vi "数据查询_数据查询_古田污水厂.vi"() -> ()   [LabVIEW 2016]
uses:
  <vilib>/Utility/miscctls.llb/LVPointTypeDef.ctl
  <vilib>/Utility/miscctls.llb/LVRowAndColumnUnsignedTypeDef.ctl
  <vilib>/addons/database/_DB Variant To Data/Database Variant To Data.xnode
panel:
  in  "工作模式":string(combo)="全部数据"
  out "连接的字符串":string
  out "选中数据表":string
  in  "查询":bool
  in  "结束日期":string="2020/01/01"
  in  "起始日期":string="2010/01/01"
  out "XY图":cluster{"data":timestamp[], "data":dbl[]}[](graph)
  in  "组合框":string(combo)
  out "数据表":string[][](table)
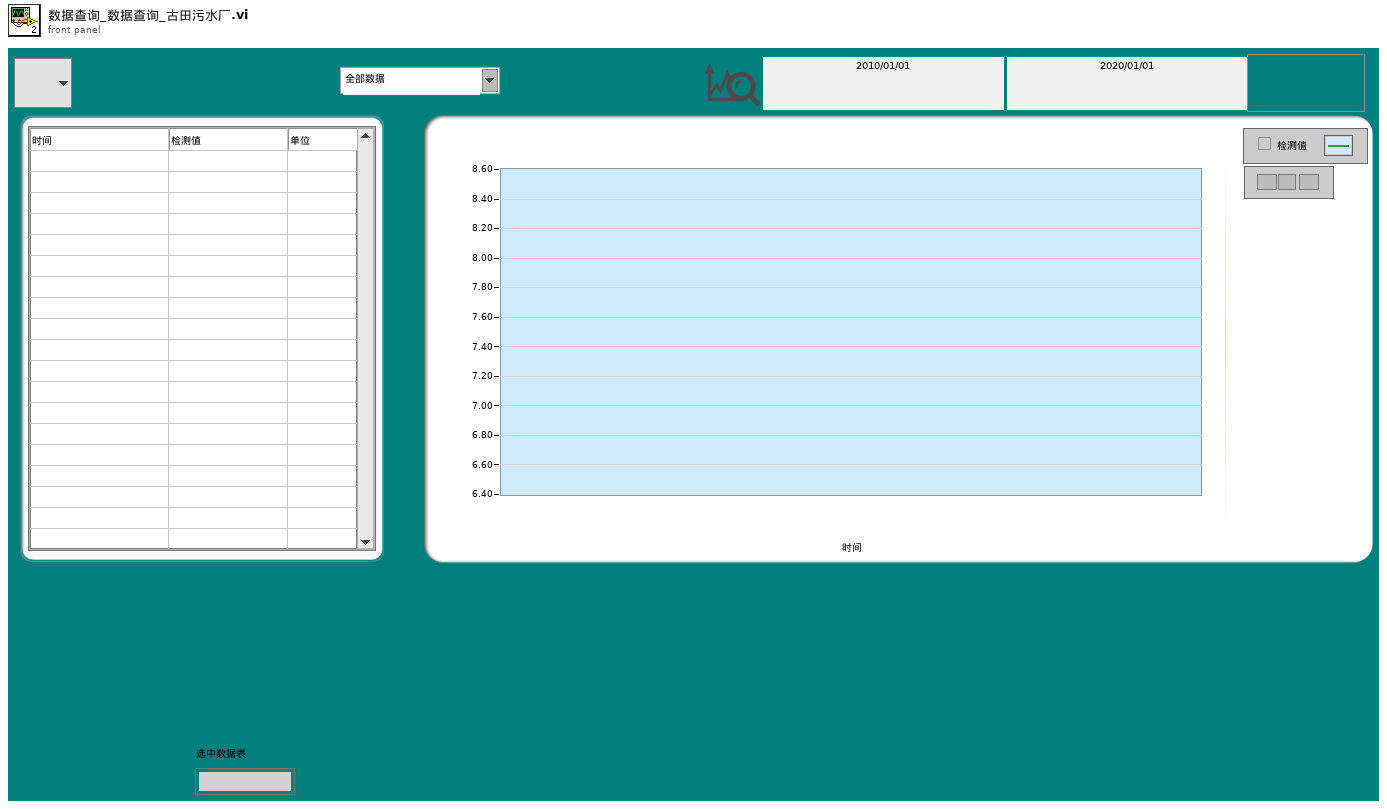
[diagram p1: front panel]
types:
  T1 = typedef "LVPointTypeDef.ctl" = cluster{"Horizontal":i16, "Vertical":i16}
  T2 = typedef "LVRowAndColumnUnsignedTypeDef.ctl" = cluster{"Row":u32, "Column":u32}
  T3 = typedef "LVPoint32TypeDef.ctl" = cluster{"Horizontal":i32, "Vertical":i32}
  T4 = typedef "LVPointDoubleTypeDef.ctl" = cluster{"Cursor X":dbl, "Cursor Y":dbl}
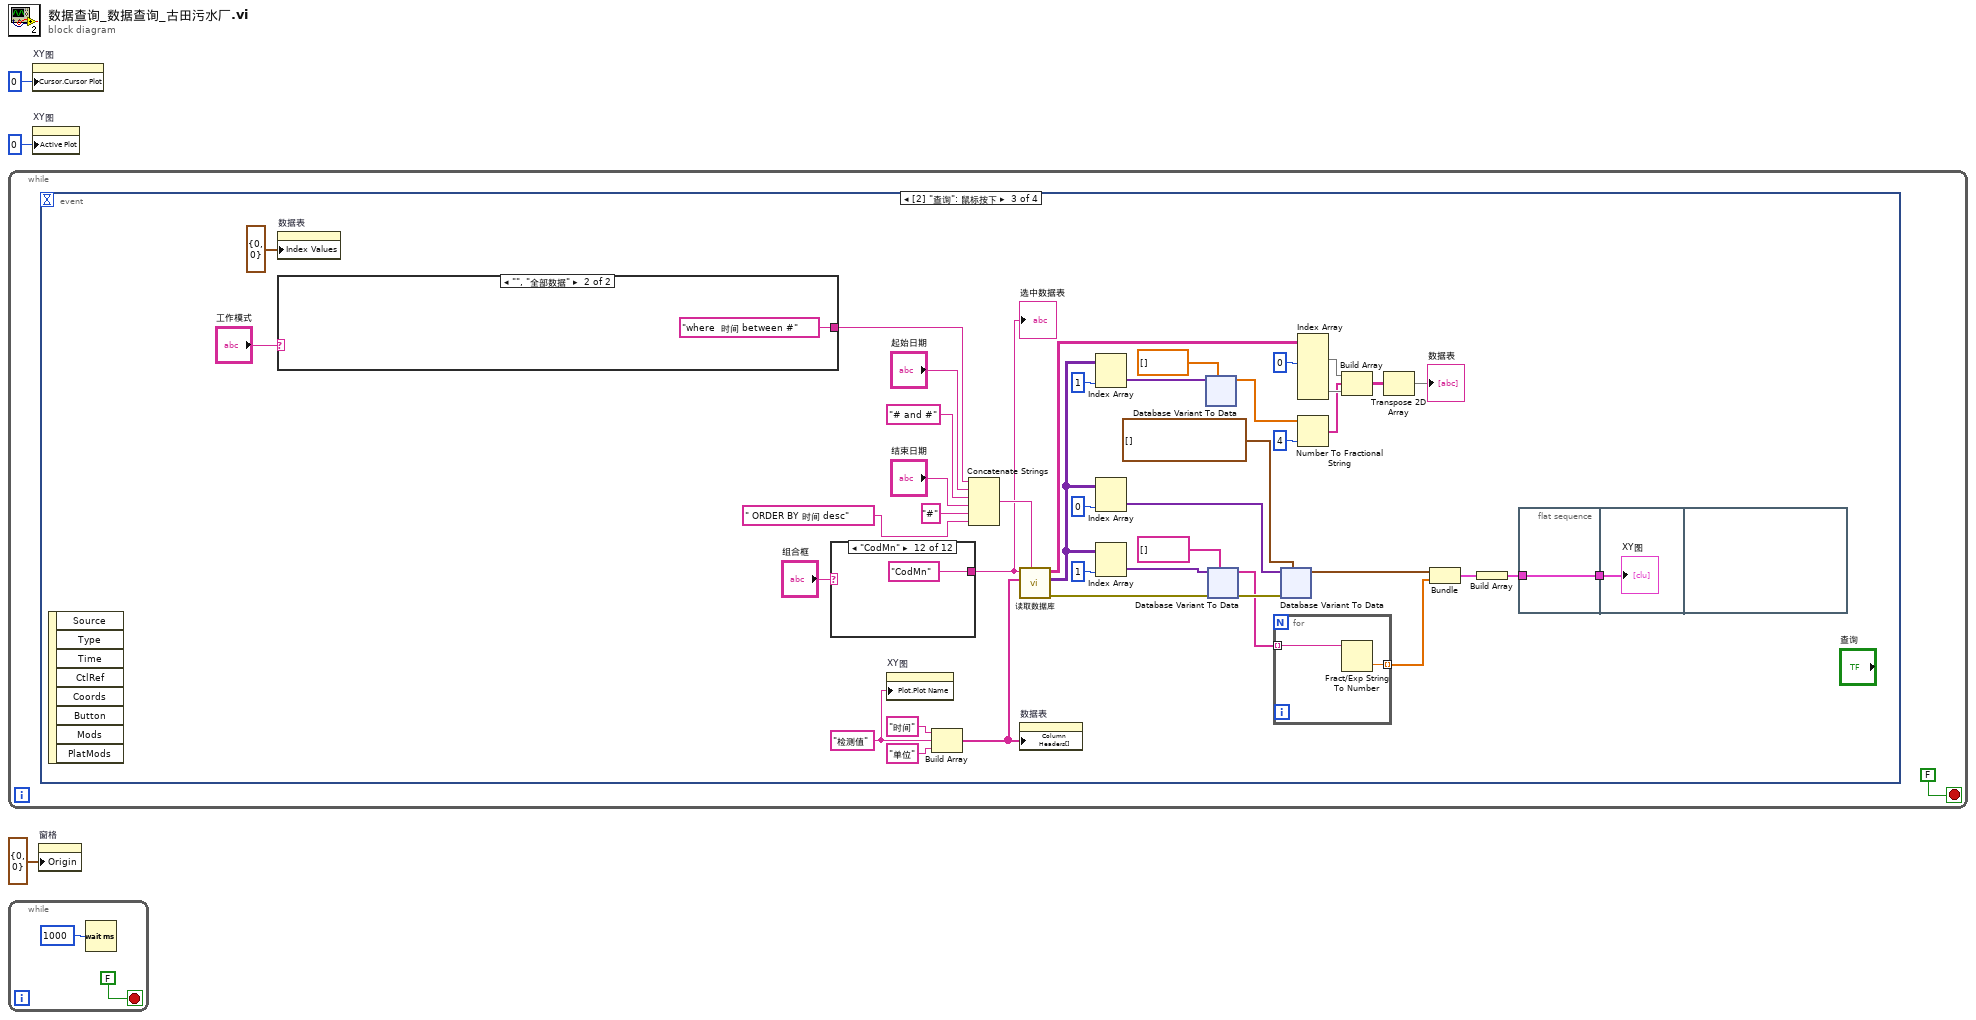
[diagram p0: block diagram]
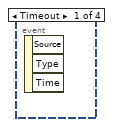
[diagram p2: hidden frame]
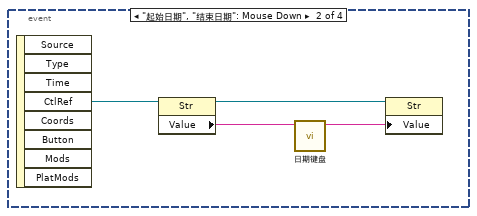
[diagram p3: hidden frame]
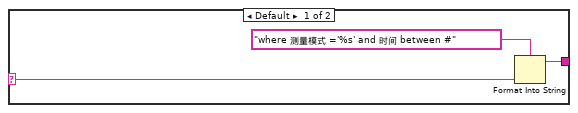
[diagram p4: hidden frame]
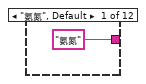
[diagram p5: hidden frame]
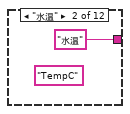
[diagram p6: hidden frame]
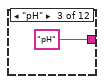
[diagram p7: hidden frame]
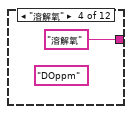
[diagram p8: hidden frame]
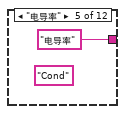
[diagram p9: hidden frame]
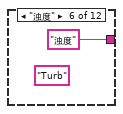
[diagram p10: hidden frame]
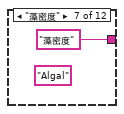
[diagram p11: hidden frame]
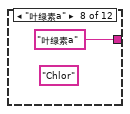
[diagram p12: hidden frame]
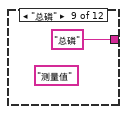
[diagram p13: hidden frame]
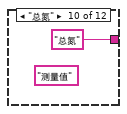
[diagram p14: hidden frame]
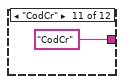
[diagram p15: hidden frame]
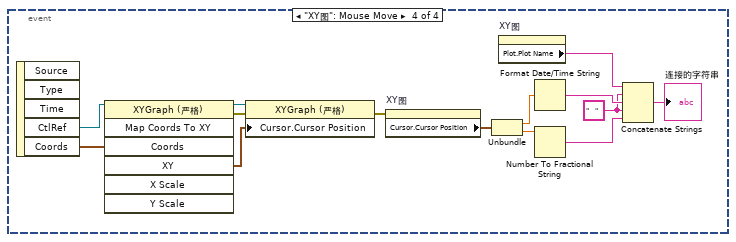
[diagram p16: hidden frame]
diagram:
  n1 = while {
    stop <- FALSE stop-if-true
    n2 = event shown="[2] \"查询\": 鼠标按下" {
      selector: _ -> [_ _ _ _]
      dyn-events: _ -> [_ _ _ _]
      timeout: _ -> [_ _ _ _]
      event Timeout {
        n3 = event-data() -> ()  [unwired: 1 in, 3 out]
      }
      event "起始日期", "结束日期": Mouse Down {
        n4 = event-data() -> ("CtlRef"=w8:refnum<vi>)  [unwired: 1 in, 7 out]
        n5 = property class="Str"(reference=w8) -> (reference out=w6:refnum<vi>, "Value"=w7:string)  [unwired: 1 in, 1 out]
        n6 = call "日期键盘.vi"("原值"=w7) -> ("x+y"=w5:string)  [unwired: 10 in]
        n7 = property class="Str"(reference=w6, "Value"=w5) -> ()  [unwired: 1 in, 2 out]
      }
      event "查询": Mouse Down {
        w22 = "检测值"
        n8 = event-data() -> ()  [unwired: 1 in, 8 out]
        n9 = property on="数据表" class="Tbl (严格)"("Index Values"=T2 {"Row"=0, "Column"=0} ("索引值")) -> ()  [unwired: 2 in, 2 out]
        n10 = case shown="\"\", \"全部数据\"" "工作模式" {
          selector: "工作模式" -> [w53 _]
          tunnel: [w51 "where  时间 between #" ("condition")] -> w10
          frame Default {
            n11 = Format Into String(format string="where 测量模式 ='%s' and 时间 between #" ("condition"), w53) -> (resulting string=w51:string)  [unwired: 2 in, 1 out]
          }
          frame "", "全部数据" {
          }
        }
        n12 = case shown="\"CodMn\"" "组合框" {
          tunnel: ["氨氮" "水温" "pH" "溶解氧" "电导率" "浊度" "藻密度" "叶绿素a" "总磷" "总氮" "CodCr" "CodMn"] -> w24
          frame "氨氮", Default {
          }
          frame "水温" {
            (unwired) "TempC"
          }
          frame "pH" {
          }
          frame "溶解氧" {
            (unwired) "DOppm"
          }
          frame "电导率" {
            (unwired) "Cond"
          }
          frame "浊度" {
            (unwired) "Turb"
          }
          frame "藻密度" {
            (unwired) "Algal"
          }
          frame "叶绿素a" {
            (unwired) "Chlor"
          }
          frame "总磷" {
            (unwired) "测量值"
          }
          frame "总氮" {
            (unwired) "测量值"
          }
          frame "CodCr" {
          }
          frame "CodMn" {
          }
        }
        "选中数据表" <- w24
        n13 = property on="XY图" class="XYGraph (严格)"("Plot.Plot Name"=w22) -> ()  [unwired: 2 in, 2 out]
        n14 = Build Array("时间", w22, "单位" ("元素")) -> (w25:string[])
        n15 = Concatenate Strings(w10, "起始日期", "# and #" ("condition"), "结束日期", "#" ("condition"), " ORDER BY 时间 desc" ("字符串")) -> (w49:string)
        n16 = call "读取数据库.vi"("condition"=w49, "显示项"=w25, "组合框"=w24) -> ("error out"=w40:errorcluster, "data"=w19:variant[][], "表格"=w32:string[][])  [unwired: 5 in, 1 out]
        n17 = property on="数据表" class="Tbl (严格)"("Column Headers[]"=w25) -> ()  [unwired: 2 in, 2 out]
        n18 = Index Array(array=w19, index (col)=1 ("禁用的索引 (列)")) -> (element=w17:variant[])  [unwired: 1 in]
        n19 = Index Array(array=w19, index (col)=0 ("禁用的索引 (列)")) -> (element=w43:variant[])  [unwired: 1 in]
        n20 = Index Array(array=w19, index (col)=1 ("禁用的索引 (列)")) -> (element=w41:variant[])  [unwired: 1 in]
        n21 = xnode "Database Variant To Data"("database variant"=w17, "type"=sgl[] []) -> ("data"=w15:sgl[])  [unwired: 1 in, 1 out]
        n22 = xnode "Database Variant To Data"("database variant"=w41, "error in (no error)"=w40, "type"=string[] []) -> ("data"=w23:string[], "error out"=w39:errorcluster)
        n23 = for {
          tunnel: w23 -> [w94] mode=indexing
          tunnel: [w93] -> w9 mode=indexing
          n24 = Fract/Exp String To Number(string=w94) -> (number=w93:dbl)  [unwired: 3 in, 1 out]
        }
        n25 = xnode "Database Variant To Data"("database variant"=w43, "error in (no error)"=w39, "type"=timestamp[] []) -> ("data"=w34:timestamp[])  [unwired: 1 out]
        n26 = Index Array(array=w32, index (col) #1=0 ("禁用的索引 (列)")) -> (element #1=w30:string[], element #3=w20:string[])  [unwired: 5 in, 1 out]
        n27 = Number To Fractional String(number=w15, precision (6)=i16 4 ("精度(6)")) -> (F-format string=w13:string[])  [unwired: 2 in]
        n28 = Build Array(w30, w13, w20) -> (w29:string[][])
        n29 = Transpose 2D Array(2D array=w29) -> (transposed array=→"数据表":string[][])
        n30 = Bundle("data"=w34, w9) -> (w35:cluster{"data":timestamp[], dbl[]})  [unwired: 1 in]
        n31 = Build Array(w35) -> (w36:cluster{"data":timestamp[], dbl[]}[])
        n32 = flat-sequence {
          tunnel: [w107] -> w37
          tunnel: w36 -> [w107]
          tunnel: w37 -> [w108]
          frame #0 {
          }
          frame #1 {
            "XY图" <- w108
          }
          frame #2 {
          }
        }
      }
      event "XY图": Mouse Move {
        w202 = "   " ("字符串")
        n33 = event-data() -> ("CtlRef"=w212:refnum<vi>, "Coords"=w211:T3)  [unwired: 1 in, 3 out]
        n34 = invoke class="XYGraph (严格)" method="Map Coords To XY"(reference=w212, "Coords"=w211) -> (reference out=w210:refnum<vi>, error out=w207:errorcluster, "XY"=w209:cluster{"X":dbl, "Y":dbl})  [unwired: 5 in, 4 out]
        n35 = property class="XYGraph (严格)"(reference=w210, error in=w207, "Cursor.Cursor Position"=w209) -> (error out=w208:errorcluster)  [unwired: 1 out]
        n36 = property on="XY图" class="XYGraph (严格)"(error in=w208) -> ("Cursor.Cursor Position"=w205:T4)  [unwired: 1 in, 2 out]
        n37 = Unbundle(w205) -> ("Cursor X"=w204:dbl, "Cursor Y"=w201:dbl)
        n38 = property on="XY图" class="XYGraph (严格)"() -> ("Plot.Plot Name"=w199:string)  [unwired: 2 in, 2 out]
        n39 = Format Date/Time String(seconds (now)=w204) -> (date/time string=w203:string)  [unwired: 2 in]
        n40 = Number To Fractional String(number=w201) -> (F-format string=w200:string)  [unwired: 3 in]
        n41 = Concatenate Strings(w199, w202, w203, w202, w200) -> (→"连接的字符串":string)
      }
    }
  }
  n42 = while {
    stop <- FALSE stop-if-true
    n43 = Wait (ms)(milliseconds to wait=u32 1000 ("等待时间（毫秒）")) -> ()  [unwired: 1 out]
  }
  n44 = property on="XY图" class="XYGraph (严格)"("Cursor.Cursor Plot"=0 ("游标.游标关联曲线")) -> ()  [unwired: 2 in, 2 out]
  n45 = property on="XY图" class="XYGraph (严格)"("Active Plot"=u32 0 ("活动曲线")) -> ()  [unwired: 2 in, 2 out]
  n46 = property on="窗格" class="Pane"("Origin"=T1 {"Horizontal"=0, "Vertical"=0} ("原点")) -> ()  [unwired: 2 in, 2 out]
